vi "Untitled 5 (SubVI).vi"(8 "pixsize":dbl, 10 "results (amplitude,center,stdv,residue,ofst)":dbl[](array[numeric]), 11 "Array in":u16[](array[numeric])) -> (0 "fit y":dbl[](array[numeric]), 1 "fit x":dbl[](array[numeric]), 2 "real y":dbl[](array[numeric]), 3 "real x":dbl[](array[numeric]))   [LabVIEW 2024]
panel:
  in  "plot points":i32=1000
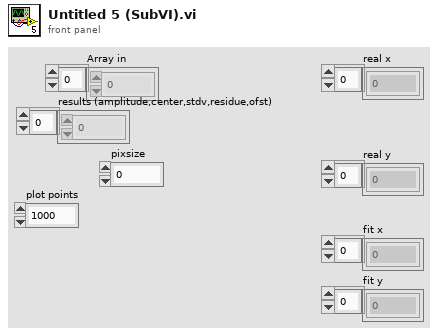
[diagram p1: front panel]
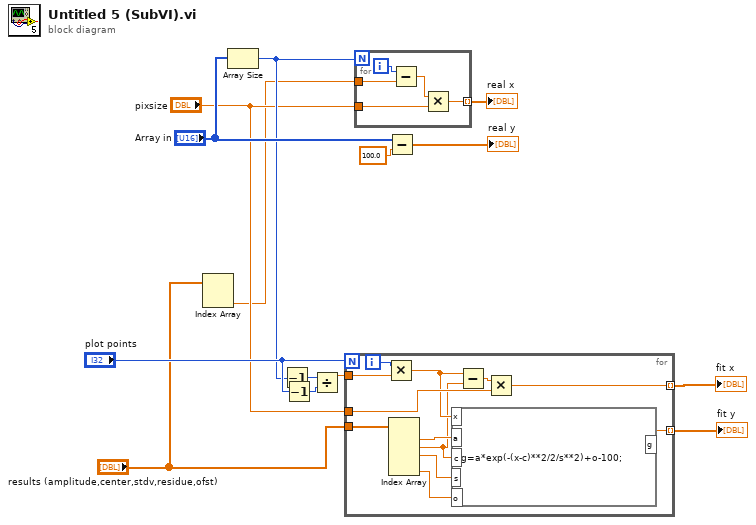
[diagram p0: block diagram]
diagram:
  n1 = Index Array(array="results (amplitude,center,stdv,residue,ofst)") -> (element #2=w1:dbl)  [unwired: 2 in, 1 out]
  n2 = Array Size(array="Array in") -> (size(s)=w4:i32)
  n3 = Decrement(x=w4) -> (x-1=w9:i32)
  n4 = Decrement(x="plot points") -> (x-1=w7:i32)
  n5 = Divide(x=w9, y=w7) -> (x/y=w8:dbl)
  n6 = for {
    N: "plot points" -> [_]
    tunnel: w8 -> [w26]
    tunnel: "results (amplitude,center,stdv,residue,ofst)" -> [w25]
    tunnel: [w21] -> w5 mode=indexing
    tunnel: "pixsize" -> [w20]
    tunnel: [w19] -> w6 mode=indexing
    i -> [w16]
    n7 = Multiply(x=w16, y=w26) -> (x*y=w17:dbl)
    n8 = Index Array(array=w25) -> (element #1=w24:dbl, element #2=w15:dbl, element #3=w23:dbl, element #5=w22:dbl)  [unwired: 5 in, 1 out]
    n9 = formula code="g=a*exp(-(x-c)**2/2/s**2)+o-100;"("a"=w24, "c"=w15, "s"=w23, "o"=w22, "x"=w17) -> ("g"=w21:dbl)
    n10 = Subtract(x=w17, y=w15) -> (x-y=w18:dbl)
    n11 = Multiply(x=w18, y=w20) -> (x*y=w19:dbl)
  }
  "fit x" <- w6
  "fit y" <- w5
  n12 = for {
    N: w4 -> [_]
    tunnel: w1 -> [w30]
    tunnel: "pixsize" -> [w28]
    tunnel: [w27] -> w12 mode=indexing
    i -> [w31]
    n13 = Subtract(x=w31, y=w30) -> (x-y=w29:dbl)
    n14 = Multiply(x=w29, y=w28) -> (x*y=w27:dbl)
  }
  "real x" <- w12
  n15 = Subtract(x="Array in", y=100.0) -> (x-y=→"real y":dbl[])
